vi "stringArray2String3.vi"(1 "字符串数组":string[](array[string])) -> (0 "字符串":string)   [LabVIEW 2018]
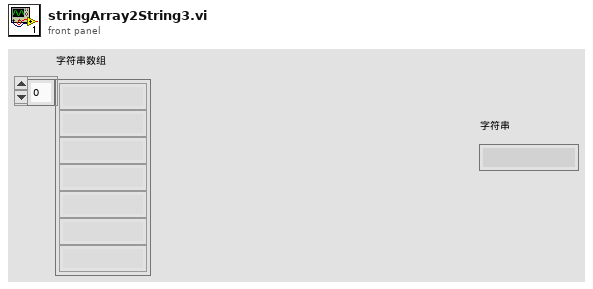
[diagram p1: front panel]
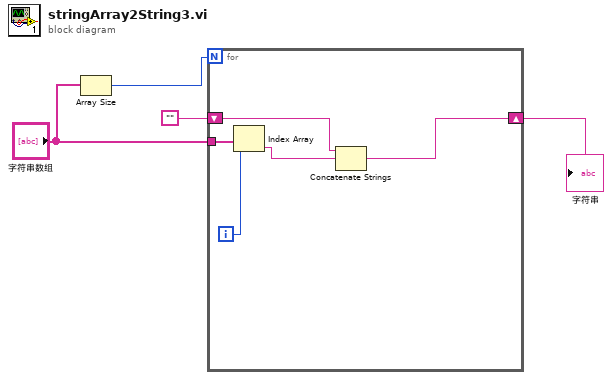
[diagram p0: block diagram]
diagram:
  n1 = Array Size(array="字符串数组") -> (size(s)=w4:i32)
  n2 = for {
    N: w4 -> [_]
    shift-right: [w9] -> w1
    shift-left: "" -> [w5]
    tunnel: "字符串数组" -> [w8]
    i -> [w7]
    n3 = Index Array(array=w8, index=w7) -> (element=w6:string)
    n4 = Concatenate Strings(w5, w6) -> (w9:string)  [unwired: 1 in]
  }
  "字符串" <- w1
